vi "solar_cfg Close.vi"(0 "Config Refnum":refnum<data-value>, 5 "Write File if Changed (T)":bool=TRUE, 7 "Write Comments? (T)":bool=TRUE, 9 "Force Dirty? (F)":bool, 11 "error in (no error)":errorcluster) -> (4 "Config Path (*.ini)":path, 15 "error out":errorcluster)   [LabVIEW 2018]
doc: "This VI closes and write to a configuration file (*.ini). Set Force Dirty to ensure the configuration file is updated. \n\n[Section]\nKey = \"Value\" #Comment"
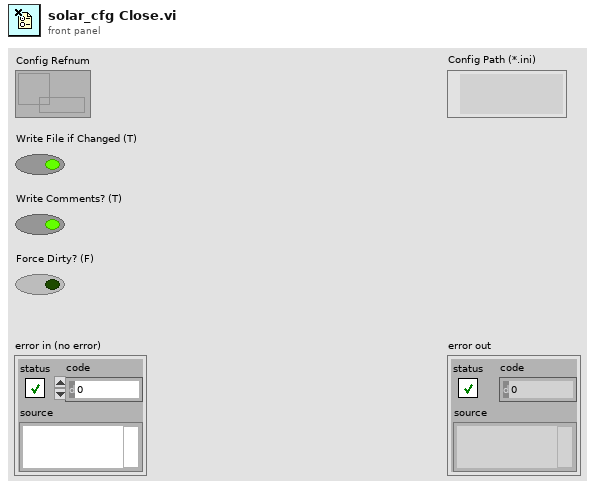
[diagram p1: front panel]
types:
  T1 = cluster{"Dirty":bool, "Semaphore":refnum<queue>, "Sections":cluster{"Section":string, "kvc":string[][]}[], "Path":path}
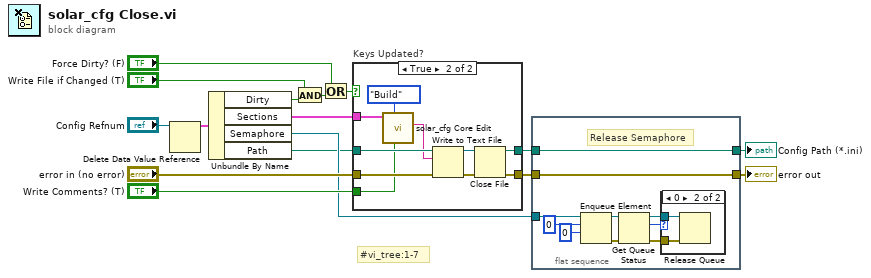
[diagram p0: block diagram]
diagram:
  # "#vi_tree:1-7"
  n1 = Delete Data Value Reference(data value reference="Config Refnum") -> (data value=w7:T1)  [unwired: 1 in, 1 out]
  n2 = Unbundle By Name(w7) -> ("Dirty"=w2:bool, "Sections"=w9:cluster{"Section":string, "kvc":string[][]}[], "Semaphore"=w8:refnum<queue>, "Path"=w6:path)
  n3 = And(x="Write File if Changed (T)", y=w2) -> (x .and. y?=w5:bool)
  n4 = Or(x="Force Dirty? (F)", y=w5) -> (x .or. y?=w4:bool)
  n5 = case "Keys Updated?" shown="True" w4 {
    tunnel: "Write Comments? (T)" -> [_ w19]
    tunnel: "error in (no error)" -> [w17 w26]
    tunnel: w6 -> [w18 w25]
    tunnel: [w18 w24] -> w11
    tunnel: [w17 w23] -> w10
    tunnel: w9 -> [_ w22]
    frame False {
    }
    frame True {
      n6 = call "solar_cfg Core Edit.vi"("Write Comments? (T)"=w19, "Action (Read)"=enum8{"Read", "Write", "Parse", "Build"}."Build", "Sections in"=w22) -> ("Value/String out"=w21:string)  [unwired: 4 in, 4 out]
      n7 = Write to Text File(file (use dialog)=w25, text=w21, error in=w26) -> (refnum out=w28:refnum<file>, error out=w27:errorcluster)  [unwired: 1 in, 1 out]
      n8 = Close File(refnum=w28, error in=w27) -> (path=w24:path, error out=w23:errorcluster)
    }
  }
  n9 = flat-sequence {
    tunnel: w8 -> [w38]
    tunnel: [w29] -> w13
    tunnel: w11 -> [w29]
    tunnel: w10 -> [w30]
    tunnel: [w30] -> w15
    frame #0 {
      # "Release Semaphore"
      n10 = Enqueue Element(queue=w38, element=u8 0, timeout in ms (-1)=0) -> (queue out=w35:refnum<queue>, error out=w34:errorcluster)  [unwired: 1 in, 1 out]
      n11 = Get Queue Status(queue=w35, error in (no error)=w34) -> (queue out=w32:refnum<queue>, # pending remove=w33:i32, error out=w31:errorcluster)  [unwired: 1 in, 5 out]
      n12 = case shown="0" w33 {
        tunnel: w32 -> [_ w40]
        tunnel: w31 -> [_ w39]
        frame Default {
        }
        frame 0 {
          n13 = Release Queue(queue=w40, error in (no error)=w39) -> ()  [unwired: 1 in, 3 out]
        }
      }
    }
  }
  "error out" <- w15
  "Config Path (*.ini)" <- w13
